vi "HaltStageOutput.vi"(1 "Image Settings":T1={"Start Position (µm)"={"x"=0.0, "y"=0.0, "z"=0.0}, "End Position (µm)"={"x"=10.0, "y"=10.0, "z"=0.0}, "Image Resolution (nm/pixel)"={"x"=50.0, "y"=50.0, "z"=100.0}, "Image Size (µm)"={"x"=10.0, "y"=10.0, "z"=0.0}, "Image Size (pixel)"={"x"=50, "y"=50, "z"=0}, "Time Resolution\n(ms/pixel)"=7.0, "1st Axis"=0, "2nd Axis"=1, "Retrace"=FALSE, "Estimated Time"=""} {"2nd Axis" items=["x", "y", "z"]; "1st Axis" items=["x", "y", "z"]; "Time Resolution\n(ms/pixel)" format="%.2f"; "Image Resolution (nm/pixel)"."z" format="%.2f"; "Image Resolution (nm/pixel)"."y" format="%.2f"; "Image Resolution (nm/pixel)"."x" format="%.2f"; "Image Size (µm)"."z" format="%.2f"; "Image Size (µm)"."y" format="%.2f"; "Image Size (µm)"."x" format="%.2f"; "End Position (µm)"."z" format="%.2f"; "End Position (µm)"."y" format="%.2f"; "End Position (µm)"."x" format="%.2f"; "Start Position (µm)"."z" format="%.2f"; "Start Position (µm)"."y" format="%.2f"; "Start Position (µm)"."x" format="%.2f"}) -> (0 "Error out":errorcluster)   [LabVIEW 2009]
uses:
  ImageSettings.ctt
panel:
  in  "Case Constant\n(See Context Help)":bool
  in  "VI Refnum":refnum<vi>
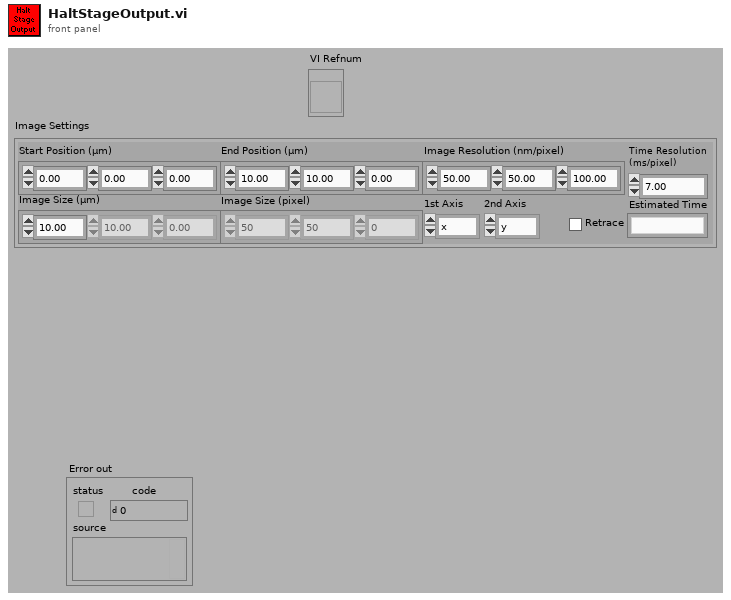
[diagram p1: front panel]
types:
  T1 = typedef "ImageSettings.ctt" = cluster{"Start Position (µm)":cluster{"x":dbl, "y":dbl, "z":dbl}, "End Position (µm)":cluster{"x":dbl, "y":dbl, "z":dbl}, "Image Resolution (nm/pixel)":cluster{"x":dbl, "y":dbl, "z":dbl}, "Image Size (µm)":cluster{"x":dbl, "y":dbl, "z":dbl}, "Image Size (pixel)":cluster{"x":u32, "y":u32, "z":u32}, "Time Resolution\n(ms/pixel)":dbl, "1st Axis":u16, "2nd Axis":u16, "Retrace":bool, "Estimated Time":string}
  T2 = enum16{"Get Type", "Set Type", "GetStageInit", "GetWriteStageSetting", "GetInitializeStageOutput", "GetSetAxisPosition", "GetSetPos", "GetSetupStage", "HaltStageOutput"}
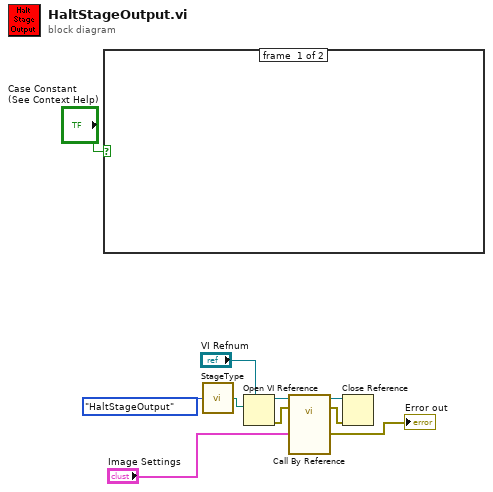
[diagram p0: block diagram]
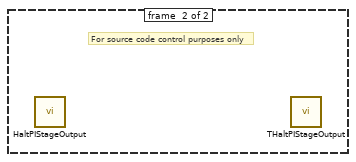
[diagram p2: hidden frame]
diagram:
  n1 = case shown="True" "Case Constant\n(See Context Help)" {
    frame #0 {
    }
    frame #1 {
      # "For source code control purposes only"
      n2 = call "HaltPIStageOutput.vi"() -> ()  [unwired: 1 in, 1 out]
      n3 = call "THaltPIStageOutput.vi"() -> ()  [unwired: 1 in, 1 out]
    }
  }
  n4 = call "StageType.vi"("Function"=T2."HaltStageOutput") -> ("VI Path"=w9:path)  [unwired: 2 in, 2 out]
  n5 = Open VI Reference(type specifier VI Refnum (for type only)="VI Refnum", vi path=w9) -> (vi reference=w8:refnum<vi>, error out=w7:errorcluster)  [unwired: 4 in]
  n6 = call-by-ref "?"(reference=w8, error in=w7, "Image Settings"="Image Settings") -> (reference out=w6:refnum<vi>, error out=w5:errorcluster, 0:"error out"=→"Error out":errorcluster)
  n7 = Close Reference(reference=w6, error in (no error)=w5) -> ()  [unwired: 1 out]
